vi "Convert Hex to FP.vi"(11 "Hex String In":string) -> (3 "Number":sgl=92.92 format="%.10f")   [LabVIEW 2014, in "Meerstetter Lib.lvlib" / "Meerstetter TEC.lvclass"]
uses:
  Meerstetter TEC.lvclass
panel:
  out "Byte Array Out":bool[](array[boolean])
  out "Exponent":i32=6
  out "Mantissa":dbl=1.4518749713897705 format="%.8f"
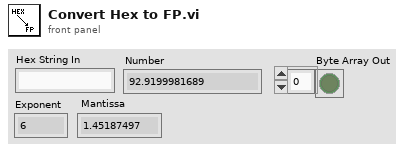
[diagram p1: front panel]
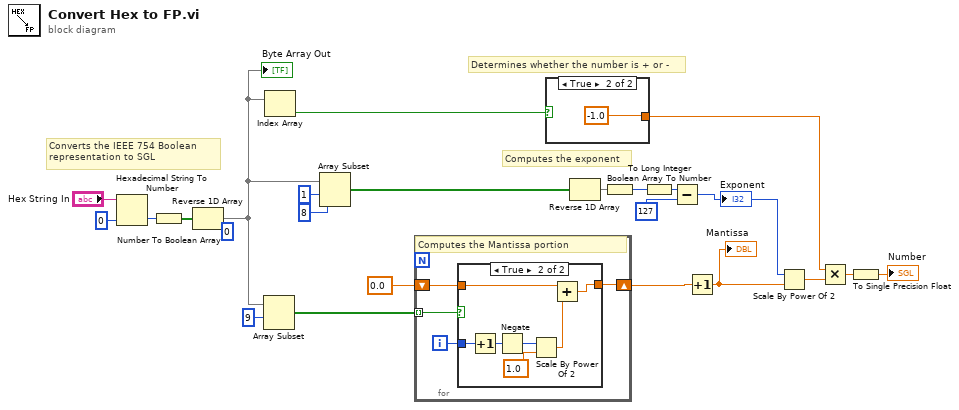
[diagram p0: block diagram]
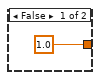
[diagram p2: hidden frame]
diagram:
  (unwired) 0 ("index")
  # "Converts the IEEE 754 Boolean \nrepresentation to SGL"
  # "Computes the exponent"
  # "Determines whether the number is + or -"
  n1 = Hexadecimal String To Number(string="Hex String In", default (0uL)=u32 0 ("default (0 U32)")) -> (number=w9:u32)  [unwired: 1 in, 1 out]
  n2 = Number To Boolean Array(number=w9) -> (Boolean array=w8:bool[])
  n3 = Reverse 1D Array(array=w8) -> (reversed array=w3:bool[])
  "Byte Array Out" <- w3
  n4 = Array Subset(array=w3, index=9) -> (w1:bool[])  [unwired: 1 in]
  n5 = Index Array(array=w3) -> (element=w7:bool)  [unwired: 1 in]
  n6 = Array Subset(array=w3, index=1, length=8) -> (w4:bool[])
  n7 = for {
    tunnel: w1 -> [w27] mode=indexing
    shift-right: [w24] -> w22
    shift-left: 0.0 -> [w25]
    i -> [w26]
    # "Computes the Mantissa portion"
    n8 = case shown="True" w27 {
      tunnel: w26 -> [_ w35]
      tunnel: w25 -> [w28 w31]
      tunnel: [w28 w29] -> w24
      frame False {
      }
      frame True {
        n9 = Increment(x=w35) -> (x+1=w34:i32)
        n10 = Negate(x=w34) -> (-x=w33:i32)
        n11 = Scale By Power Of 2(n=w33, x=1.0) -> (x*2^n=w30:dbl)
        n12 = Add(x=w31, y=w30) -> (x+y=w29:dbl)
      }
    }
  }
  n13 = case shown="True" w7 {
    tunnel: [1.0 -1.0] -> w16
    frame False {
    }
    frame True {
    }
  }
  n14 = Reverse 1D Array(array=w4) -> (reversed array=w18:bool[])
  n15 = Boolean Array To Number(Boolean array=w18) -> (number=w14:u32)
  n16 = To Long Integer(number=w14) -> (32bit integer=w13:i32)
  n17 = Subtract(x=w13, y=127) -> (x-y=w15:i32)
  "Exponent" <- w15
  n18 = Increment(x=w22) -> (x+1=w20:dbl)
  "Mantissa" <- w20
  n19 = Scale By Power Of 2(n=w15, x=w20) -> (x*2^n=w19:dbl)
  n20 = Multiply(x=w16, y=w19) -> (x*y=w17:dbl)
  n21 = To Single Precision Float(number=w17) -> (single precision float=→"Number":sgl)
